vi "detect change dir.vi"(7 "reset":bool, 9 "cont stop":u32, 10 "max dont change":i32=200, 11 "in":i32) -> (0 "x-y":i32, 1 "dont change count":i32, 2 "count":u32, 3 "change direction":bool, 4 "stop":bool)   [LabVIEW 2019, in "NeedleValve.lvclass"]
uses:
  NeedleValve.lvclass
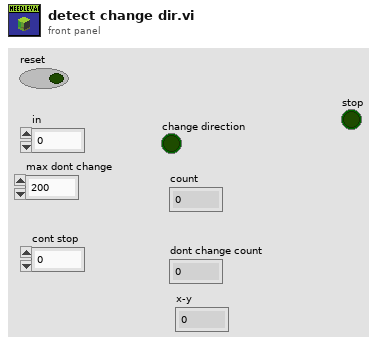
[diagram p1: front panel]
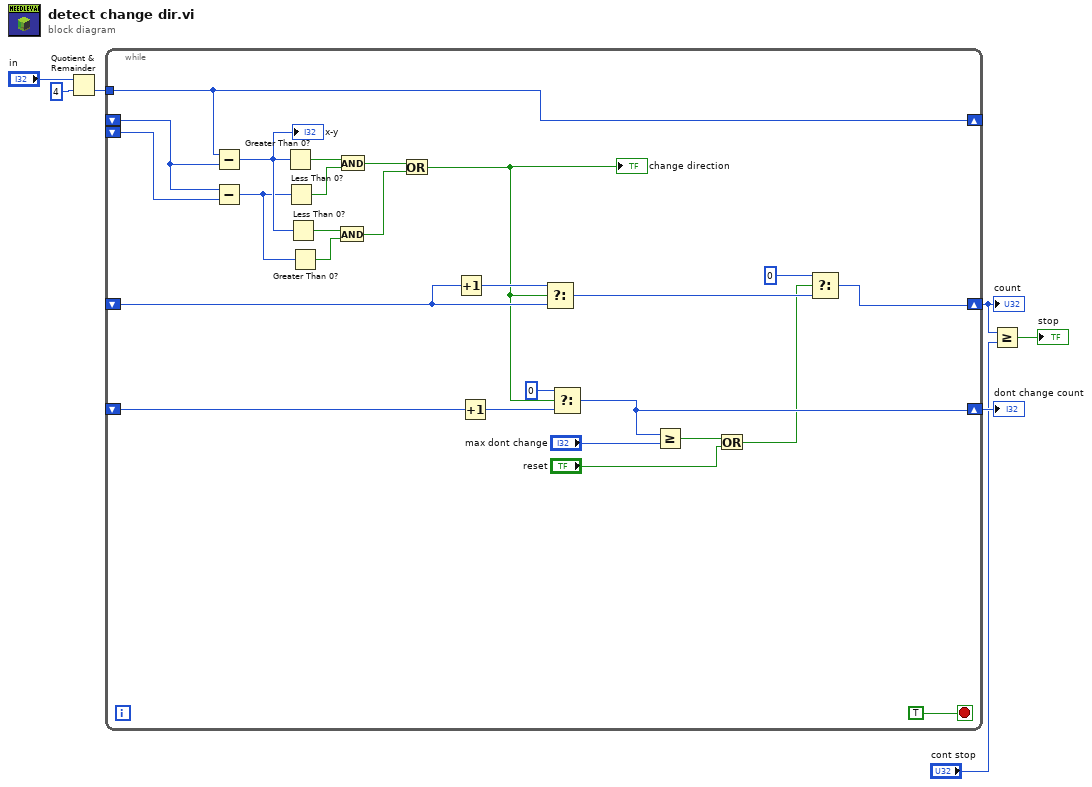
[diagram p0: block diagram]
diagram:
  n1 = Quotient & Remainder(x="in", y=4) -> (floor(x/y)=w4:i32)  [unwired: 1 out]
  n2 = while {
    shift-right: [w8] -> _
    shift-left: _ -> [w32]
    shift-left: _ -> [w31]
    shift-right: [w11] -> w3
    shift-left: _ -> [w30]
    shift-right: [w16] -> w7
    shift-left: _ -> [w27]
    tunnel: w4 -> [w8]
    stop <- TRUE stop-if-true
    n3 = Subtract(x=w8, y=w32) -> (x-y=w23:i32)
    "x-y" <- w23
    n4 = Subtract(x=w32, y=w31) -> (x-y=w22:i32)
    n5 = Greater Than 0?(x=w23) -> (x > 0?=w25:bool)
    n6 = Less Than 0?(x=w22) -> (x < 0?=w24:bool)
    n7 = Less Than 0?(x=w23) -> (x < 0?=w21:bool)
    n8 = Greater Than 0?(x=w22) -> (x > 0?=w20:bool)
    n9 = And(x=w21, y=w20) -> (x .and. y?=w18:bool)
    n10 = And(x=w25, y=w24) -> (x .and. y?=w19:bool)
    n11 = Or(x=w19, y=w18) -> (x .or. y?=w17:bool)
    "change direction" <- w17
    n12 = Increment(x=w30) -> (x+1=w29:u32)
    n13 = Increment(x=w27) -> (x+1=w26:i32)
    n14 = Select(t=w29, s=w17, f=w30) -> (s? t:f=w14:u32)
    n15 = Select(t=0, s=w17, f=w26) -> (s? t:f=w16:i32)
    n16 = Greater Or Equal?(x=w16, y="max dont change") -> (x >= y?=w12:bool)
    n17 = Or(x=w12, y="reset") -> (x .or. y?=w10:bool)
    n18 = Select(t=u32 0, s=w10, f=w14) -> (s? t:f=w11:u32)
  }
  "count" <- w3
  "dont change count" <- w7
  n19 = Greater Or Equal?(x=w3, y="cont stop") -> (x >= y?=→"stop":bool)
